vi "2L21_SPOP_estime_de_s.vi"(1 "N":u32, 2 "n":u32, 3 "s":dbl) -> (0 "S pop estimé":dbl)   [LabVIEW 2010, in "lv_02.lvlib"]
doc: "Ce Vi calcule l'écart-type estimé à partir de l'écart-type s d'un échantillon de taille n issu d'une population de taille N.\nSi la population est de taille infinie ou grande devant n, laisser la valeur 0 (par défaut)"
uses:
  lv_02.lvlib
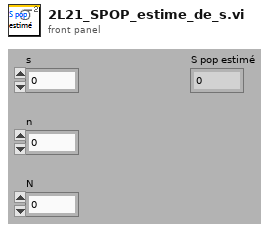
[diagram p1: front panel]
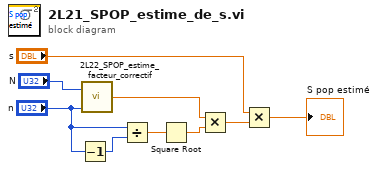
[diagram p0: block diagram]
diagram:
  n1 = Decrement(x="n") -> (x-1=w4:u32)
  n2 = call "2L22_SPOP_estime_facteur_correctif.vi"("Taille de l'échantillon"="n", "Taille population"="N") -> ("facteur S"=w5:dbl)
  n3 = Divide(x="n", y=w4) -> (x/y=w3:dbl)
  n4 = Square Root(x=w3) -> (sqrt(x)=w2:dbl)
  n5 = Multiply(x=w5, y=w2) -> (x*y=w7:dbl)
  n6 = Multiply(x="s", y=w7) -> (x*y=→"S pop estimé":dbl)
